vi "move_stp_Motion.vi"(8 "error in (no error)":errorcluster caption="错误输入（无错误）", 10 "stp":dbl min=0.0, 11 "OneMotion 输入":refnum<class "OneMotion.lvclass">) -> (0 "error out":errorcluster caption="错误输出", 3 "OneMotion 输出":refnum<class "OneMotion.lvclass">)   [LabVIEW 2016, in "MotionControl_UFO_3DOF.lvlib" / "OneMotion.lvclass"]
uses:
  <userlib>/MotionControl_UFO_3DOF/OneMotion/OneMotion.lvclass
  <userlib>/MotionControl_UFO_3DOF/OneMotion/hard limit option.ctl
  <userlib>/MotionControl_UFO_3DOF/OneMotion/OneMotion.lvclass/OneMotion.ctl
  <userlib>/MotionControl_UFO_3DOF/StepMotor/StepMotor.lvclass
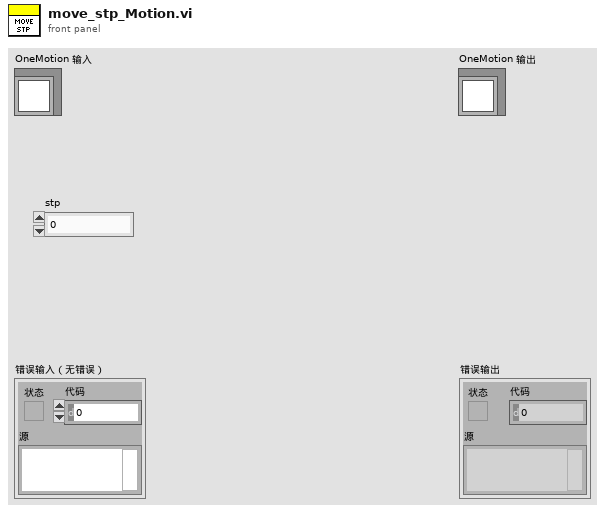
[diagram p1: front panel]
types:
  T1 = typedef "MotionControl_UFO_3DOF.lvlib/OneMotion.lvclass/hard limit option.ctl" = enum16{"STOP, and a 0.5s timeout constraint in move", "STOP, and move disabled"}
  T2 = typedef "MotionControl_UFO_3DOF.lvlib/OneMotion.lvclass/unit mode.ctl" = enum16{"motor (pulse)", "linear (mm) or radial (degree)"}
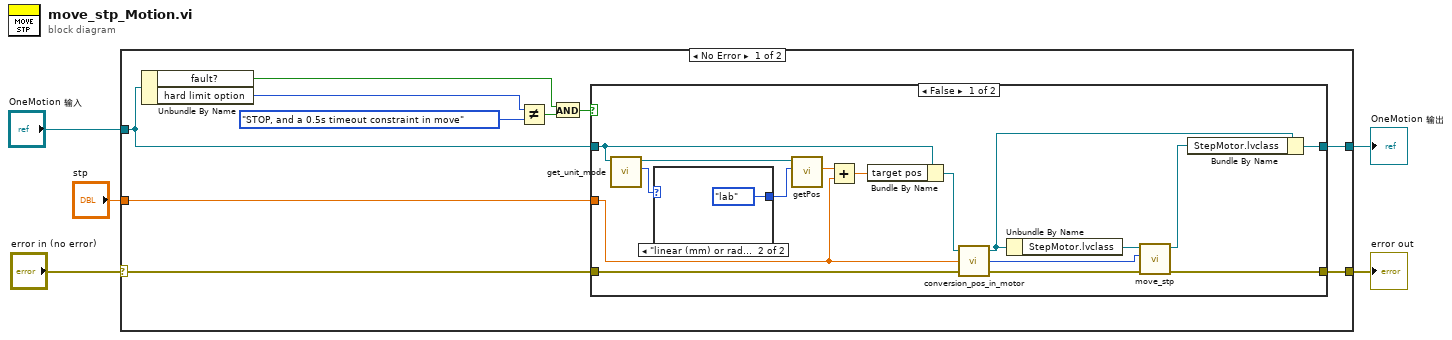
[diagram p0: block diagram]
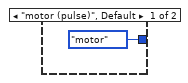
[diagram p2: hidden frame]
diagram:
  n1 = case shown="No Error" "error in (no error)" {
    selector: "error in (no error)" -> [w15 w37]
    tunnel: [w14 w37] -> w3
    tunnel: [w13 w36] -> w2
    tunnel: "OneMotion 输入" -> [w12 w36]
    tunnel: "stp" -> [w11 _]
    frame No Error {
      n2 = Unbundle By Name(w12) -> ("fault?"=w8:bool, "hard limit option"=w7:T1)
      n3 = Not Equal?(x=w7, y=hard_limit_option."STOP, and a 0.5s timeout constraint in move" ("hard limit option")) -> (x != y?=w9:bool)
      n4 = And(x=w8, y=w9) -> (x .and. y?=w6:bool)
      n5 = case shown="False" w6 {
        tunnel: w15 -> [w31 w34]
        tunnel: [w25 w34] -> w14
        tunnel: w11 -> [w17 _]
        tunnel: [w28 w35] -> w13
        tunnel: w12 -> [w22 w35]
        frame False {
          n6 = call-dynamic "get_unit_mode.vi"("OneMotion输入"=w22) -> ("unit mode"=w20:T2, "OneMotion输出"=w21:refnum<class "OneMotion.lvclass">)  [unwired: 8 in, 1 out]
          n7 = case shown="\"linear (mm) or radial (degree)\"" w20 {
            tunnel: [enum16{"lab", "motor"}."motor" ("lab or motor") enum16{"lab", "motor"}."lab" ("lab or motor")] -> w19
            frame "motor (pulse)", Default {
            }
            frame "linear (mm) or radial (degree)" {
            }
          }
          n8 = call <userlib>:"getPos.vi"("lab or motor"=w19, "OneMotion 输入"=w21) -> ("pos"=w18:dbl)  [unwired: 7 in, 2 out]
          n9 = Add(x=w18, y=w17) -> (x+y=w16:dbl)
          n10 = Bundle By Name(cluster=w22, "target pos"=w16) -> (w29:refnum<class "OneMotion.lvclass">)
          n11 = call <userlib>:"conversion_pos_in_motor.vi"("error in (no error)"=w31, "pos"=w17, "OneMotion 输入"=w29) -> ("error out"=w26:errorcluster, "pos in motor"=w23:i32, "OneMotion 输出"=w30:refnum<class "OneMotion.lvclass">)
          n12 = Unbundle By Name(w30) -> ("StepMotor.lvclass"=w27:refnum<class "StepMotor.lvclass">)
          n13 = call <userlib>:"move_stp.vi"("error in (no error)"=w26, "stp"=w23, "StepMotor 输入"=w27) -> ("error out"=w25:errorcluster, "StepMotor 输出"=w24:refnum<class "StepMotor.lvclass">)  [unwired: 7 in]
          n14 = Bundle By Name(cluster=w30, "StepMotor.lvclass"=w24) -> (w28:refnum<class "OneMotion.lvclass">)
        }
        frame True {
        }
      }
    }
    frame Error {
    }
  }
  "error out" <- w3
  "OneMotion 输出" <- w2
